vi "LCP Get Drive Pos Cnt.vi"(8 "error in (no error)":errorcluster caption="Fehler (Eingang, kein Fehler)", 11 "Pump Handle":i64) -> (0 "error out":errorcluster caption="Fehler (Ausgang)", 3 "Position Counter":i32)   [LabVIEW 2021, in "labbCAN_Pump_API.lvlib"]
doc: "LCP_Func long LCP_CALL LCP_GetDrivePosCnt(dev_hdl hPump, long *pPosCntValue);"
uses:
  labbCAN_Pump_API.lvlib
  labbCAN_Pump_API.dll
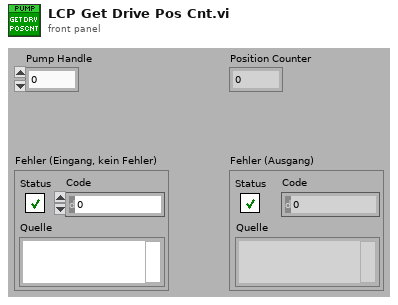
[diagram p1: front panel]
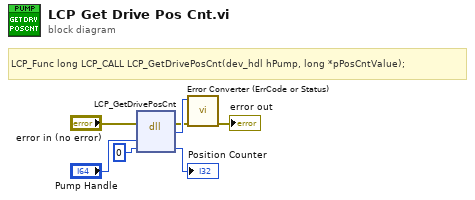
[diagram p0: block diagram]
diagram:
  # "LCP_Func long LCP_CALL LCP_GetDrivePosCnt(dev_hdl hPump, long *pPosCntValue);"
  n1 = dll-call lib="C:/Users/olaja/AppData/Local/CETONI_SDK/labbCAN_Pump_API.*" fn="LCP_GetDrivePosCnt"(error in="error in (no error)", "hPump"="Pump Handle", "pPosCntValue"=0) -> (error out=w2:errorcluster, "Rückgabetyp"=w3:i32, "pPosCntValue"=→"Position Counter":i32)  [unwired: 3 in, 1 out]
  n2 = call "Error Converter (ErrCode or Status).vi"("error in (no error)"=w2, "error code"=w3) -> ("error out"=→"error out":errorcluster)  [unwired: 9 in]
